vi "Functional data-Save.vi"(8 "error in":errorcluster, 9 "Reshaped Array":u32[][](array[numeric]), 10 "ROI Save interface cluster":T1, 11 "Data folder path":path=path "C:/") -> (0 "error out":errorcluster)   [LabVIEW 2017]
uses:
  User Interface/Visualisation/Functional Imaging Viewer/Typedefs/ROI Save interface cluster.ctl
  <userlib>/My Palettes.lib/Files & paths/Spreadsheet/Write To Spreadsheet File (I64)-Mod.vi
  User Interface/Visualisation/Functional Imaging Viewer/xcontrol/XGrapher.xctl
panel:
  out "File path & name":path
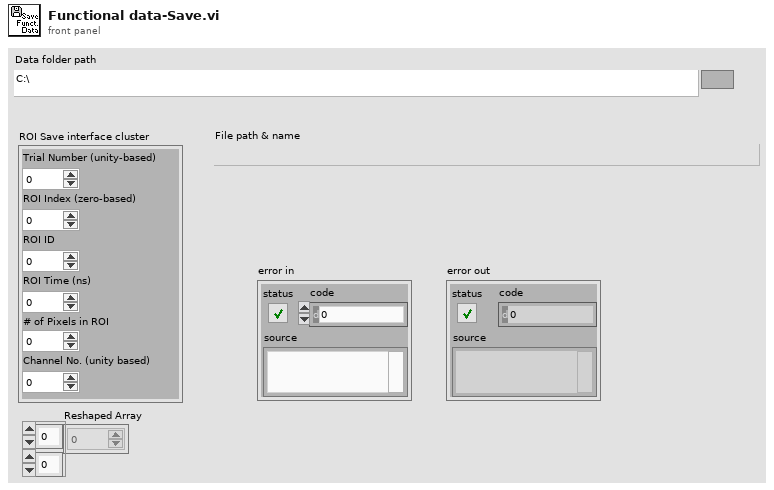
[diagram p1: front panel]
types:
  T1 = typedef "ROI Save interface cluster.ctl" = cluster{"Trial Number (unity-based)":i32, "ROI Index (zero-based)":i32, "ROI ID":i32, "ROI Time (ns)":i32, "# of Pixels in ROI":i32, "Channel No. (unity based)":i32}
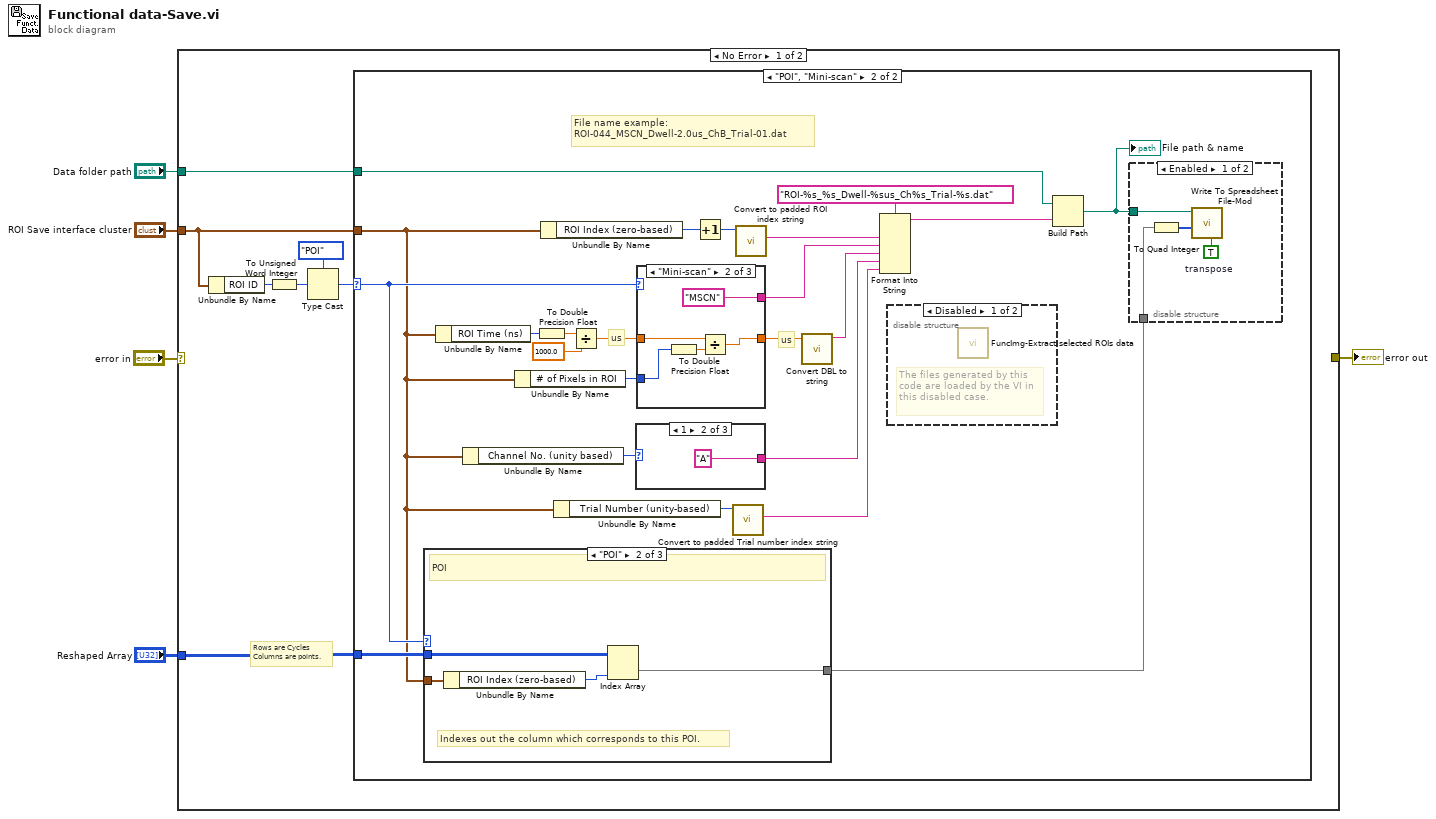
[diagram p0: block diagram]
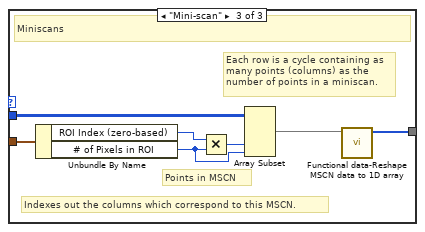
[diagram p4: hidden frame]
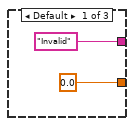
[diagram p7: hidden frame]
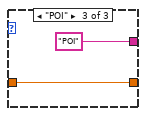
[diagram p8: hidden frame]
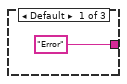
[diagram p9: hidden frame]
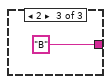
[diagram p10: hidden frame]
diagram:
  n1 = case shown="No Error" "error in" {
    selector: "error in" -> [_ w63]
    tunnel: "Data folder path" -> [w12 _]
    tunnel: "ROI Save interface cluster" -> [w8 _]
    tunnel: "Reshaped Array" -> [w6 _]
    tunnel: [_ w63] -> w1
    frame No Error {
      # "Rows are Cycles\nColumns are points."
      n2 = Unbundle By Name(w8) -> ("ROI ID"=w11:i32)
      n3 = To Unsigned Word Integer(number=w11) -> (unsigned 16bit integer=w9:u16)
      n4 = Type Cast(type=enum16{"POI", "Mini-scan"}."POI" ("Type"), x=w9) -> (*(type *) &x=w7:enum16{"POI", "Mini-scan"})
      n5 = case shown="\"POI\", \"Mini-scan\"" w7 {
        selector: w7 -> [_ w17]
        tunnel: w12 -> [_ w35]
        tunnel: w8 -> [_ w15]
        tunnel: w6 -> [_ w16]
        frame Default {
          # "Invalid ROI ID"
        }
        frame "POI", "Mini-scan" {
          # "us"
          # "us"
          # "File name example:\nROI-044_MSCN_Dwell-2.0us_ChB_Trial-01.dat"
          n6 = case shown="\"POI\"" w17 {
            tunnel: w16 -> [_ w39 w44]
            tunnel: [_ w38 w45] -> w13
            tunnel: w15 -> [_ w37 w46]
            frame Default {
              # "Invalid"
            }
            frame "POI" {
              # "Indexes out the column which corresponds to this POI."
              # "POI"
              n7 = Unbundle By Name(w37) -> ("ROI Index (zero-based)"=w36:i32)
              n8 = Index Array "Index Array"(array=w39, index (col)=w36) -> (element=w38:u32[])  [unwired: 1 in]
            }
            frame "Mini-scan" {
              # "Each row is a cycle containing as many points (columns) as the number of points in a miniscan."
              # "Points in MSCN"
              # "Indexes out the columns which correspond to this MSCN."
              # "Miniscans"
              n9 = Unbundle By Name(w46) -> ("ROI Index (zero-based)"=w42:i32, "# of Pixels in ROI"=w40:i32)
              n10 = Multiply(x=w42, y=w40) -> (x*y=w41:i32)
              n11 = Array Subset(array=w44, index (col)=w41, length (col)=w40) -> (w43:u32[][])  [unwired: 2 in]
              n12 = call "Functional data-Reshape MSCN data to 1D array.vi"("Single miniscan single trial data"=w43) -> ("Reshaped array (1D)"=w45:u32[])  [unwired: 10 in]
            }
          }
          n13 = Unbundle By Name(w15) -> ("ROI Time (ns)"=w21:i32)
          n14 = Unbundle By Name(w15) -> ("Channel No. (unity based)"=w19:i32)
          n15 = Unbundle By Name(w15) -> ("# of Pixels in ROI"=w20:i32)
          n16 = To Double Precision Float(number=w21) -> (double precision float=w28:dbl)
          n17 = Unbundle By Name(w15) -> ("ROI Index (zero-based)"=w22:i32)
          n18 = Unbundle By Name(w15) -> ("Trial Number (unity-based)"=w18:i32)
          n19 = Divide(x=w28, y=1000.0) -> (x/y=w26:dbl)
          n20 = case shown="1" w19 {
            tunnel: ["Error" "A" "B"] -> w29
            frame Default {
            }
            frame 1 {
            }
            frame 2 {
            }
          }
          n21 = case shown="\"Mini-scan\"" w17 {
            tunnel: ["Invalid" ("input 1") "MSCN" ("input 1") "POI" ("input 1")] -> w31
            tunnel: w26 -> [_ w56 w58]
            tunnel: [0.0 w53 w58] -> w25
            tunnel: w20 -> [_ w55 _]
            frame Default {
            }
            frame "Mini-scan" {
              n22 = To Double Precision Float(number=w55) -> (double precision float=w54:dbl)
              n23 = Divide(x=w56, y=w54) -> (x/y=w53:dbl)
            }
            frame "POI" {
            }
          }
          n24 = Increment(x=w22) -> (x+1=w14:i32)
          n25 = call "Convert to padded Trial number index string.vi"("Trial number (unity-based)"=w18) -> ("Trial number string padded with zeroes"=w23:string)  [unwired: 10 in]
          n26 = call "Convert to padded ROI index string.vi"("ROI number"=w14) -> ("ROI index string padded with zeroes"=w32:string)  [unwired: 10 in]
          n27 = call "Convert DBL to string.vi"("DBL Value"=w25) -> ("Converted to String"=w24:string)  [unwired: 10 in]
          n28 = Format Into String(format string="ROI-%s_%s_Dwell-%sus_Ch%s_Trial-%s.dat" ("pattern"), w32, w31, w24, w29, w23) -> (resulting string=w30:string)  [unwired: 2 in, 1 out]
          n29 = disable-structure shown="Disabled" {
            frame Disabled {
              # "The files generated by this code are loaded by the VI in this disabled case."
              n30 = call "FuncImg-Extract selected ROIs data.vi"() -> ()  [unwired: 6 in, 6 out]
            }
            frame Enabled {
            }
          }
          n31 = Build Path(base path=w35, name or relative path=w30) -> (appended path=w34:path)
          "File path & name" <- w34
          n32 = disable-structure shown="Enabled" {
            disable-tunnel: w34 -> [w50 _]
            disable-tunnel: w13 -> [w47 _]
            frame Enabled {
              w49 = TRUE  # transpose
              n33 = To Quad Integer(1:w47) -> (0:w48:i64[])
              n34 = call-poly <userlib>:"Write To Spreadsheet File-Mod.vi"("transpose? (no:F)"=w49, "1D data"=w48, "file path (dialog if empty)"=w50) -> ()  [unwired: 7 in, 2 out]
            }
            frame Disabled {
            }
          }
        }
      }
    }
    frame Error {
    }
  }
  "error out" <- w1
